vi "Flipping the Ramans for 3.0.vi"(0 "Folder Name":string, 1 "Name of File":string, 2 "Timepoints":dbl[](array[numeric]), 3 "Vx array":dbl, 4 "Vy array":dbl) -> ()   [LabVIEW 2015]
uses:
  <vilib>/Utility/file.llb/Read Delimited Spreadsheet (DBL).vi
  <vilib>/Utility/file.llb/Write Delimited Spreadsheet (DBL).vi
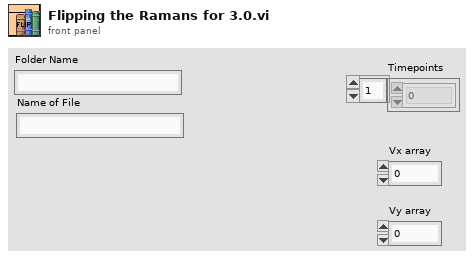
[diagram p1: front panel]
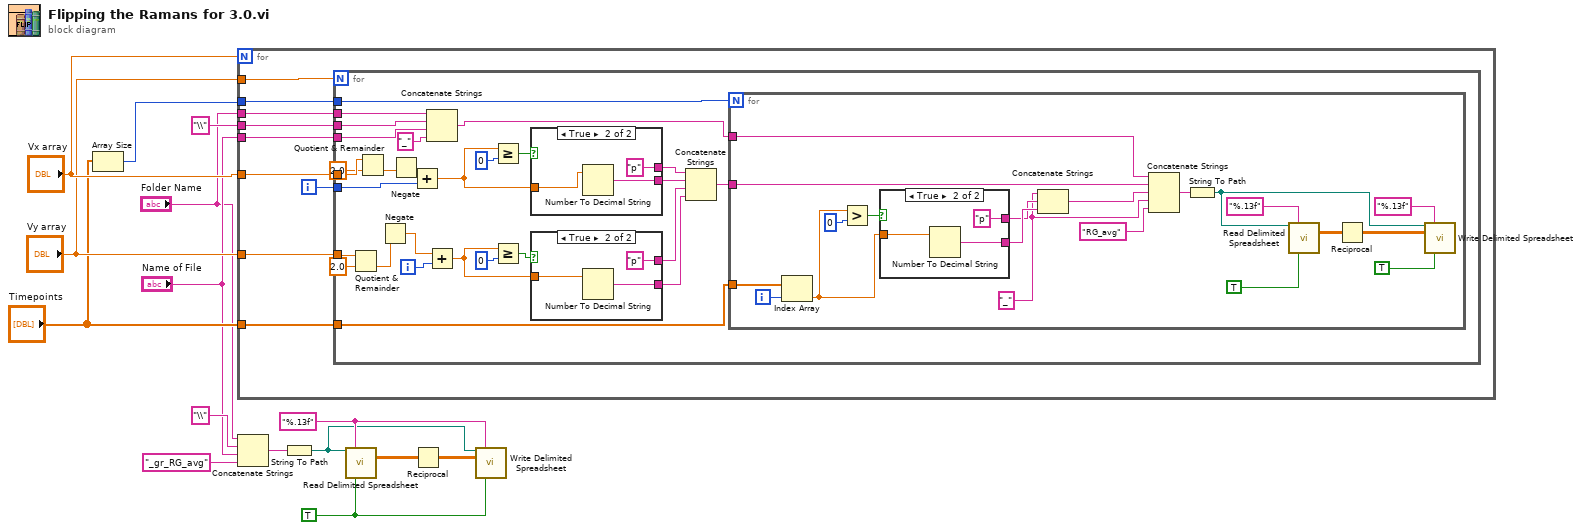
[diagram p0: block diagram]
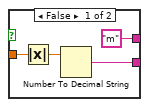
[diagram p2: hidden frame]
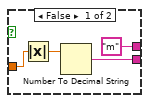
[diagram p3: hidden frame]
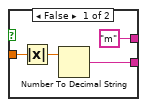
[diagram p4: hidden frame]
diagram:
  w3 = "%.13f" ("format (%.3f)")
  w2 = TRUE ("transpose? (F)")
  n1 = Array Size(array="Timepoints") -> (size(s)=w14:i32)
  n2 = for {
    N: "Vx array" -> [_]
    tunnel: "Name of File" -> [w24]
    tunnel: "\\" -> [w23]
    tunnel: "Folder Name" -> [w22]
    tunnel: "Vy array" -> [w21]
    tunnel: w14 -> [w20]
    tunnel: "Vx array" -> [w19]
    tunnel: "Vy array" -> [w17]
    tunnel: "Timepoints" -> [w16]
    i -> [w18]
    n3 = for {
      N: w21 -> [_]
      tunnel: w24 -> [w33]
      tunnel: w23 -> [w34]
      tunnel: w22 -> [w52]
      tunnel: w20 -> [w51]
      tunnel: w19 -> [w32]
      tunnel: w18 -> [w48]
      tunnel: w17 -> [w30]
      tunnel: w16 -> [w38]
      i -> [w43]
      n4 = Quotient & Remainder(x=w30, y=2.0) -> (floor(x/y)=w25:dbl)  [unwired: 1 out]
      n5 = Quotient & Remainder(x=w32, y=2.0) -> (floor(x/y)=w28:dbl)  [unwired: 1 out]
      n6 = Negate(x=w25) -> (-x=w26:dbl)
      n7 = Negate(x=w28) -> (-x=w27:dbl)
      n8 = Add(x=w27, y=w48) -> (x+y=w47:dbl)
      n9 = Concatenate Strings(w52, w34, w33, "_") -> (w36:string)
      n10 = Add(x=w26, y=w43) -> (x+y=w44:dbl)
      n11 = Greater Or Equal?(x=w47, y=0) -> (x >= y?=w49:bool)
      n12 = Greater Or Equal?(x=w44, y=0) -> (x >= y?=w46:bool)
      n13 = case shown="True" w49 {
        tunnel: ["m" "p"] -> w42
        tunnel: w47 -> [w62 w64]
        tunnel: [w60 w65] -> w41
        frame False {
          n14 = Absolute Value(x=w62) -> (abs(x)=w61:dbl)
          n15 = Number To Decimal String(number=w61) -> (decimal integer string=w60:string)  [unwired: 1 in]
        }
        frame True {
          n16 = Number To Decimal String(number=w64) -> (decimal integer string=w65:string)  [unwired: 1 in]
        }
      }
      n17 = case shown="True" w46 {
        tunnel: ["m" "p"] -> w40
        tunnel: w44 -> [w55 w57]
        tunnel: [w53 w58] -> w39
        frame False {
          n18 = Absolute Value(x=w55) -> (abs(x)=w54:dbl)
          n19 = Number To Decimal String(number=w54) -> (decimal integer string=w53:string)  [unwired: 1 in]
        }
        frame True {
          n20 = Number To Decimal String(number=w57) -> (decimal integer string=w58:string)  [unwired: 1 in]
        }
      }
      n21 = Concatenate Strings(w42, w41, w40, w39) -> (w35:string)
      n22 = for {
        N: w51 -> [_]
        tunnel: w38 -> [w83]
        tunnel: w36 -> [w74]
        tunnel: w35 -> [w73]
        i -> [w82]
        w72 = "_"
        n23 = Index Array(array=w83, index=w82) -> (element=w85:dbl)
        n24 = Greater?(x=w85, y=0) -> (0:w84:bool)
        n25 = case shown="True" w84 {
          tunnel: ["m" "p"] -> w80
          tunnel: w85 -> [w89 w91]
          tunnel: [w87 w92] -> w81
          frame False {
            n26 = Absolute Value(x=w89) -> (abs(x)=w88:dbl)
            n27 = Number To Decimal String(number=w88) -> (decimal integer string=w87:string)  [unwired: 1 in]
          }
          frame True {
            n28 = Number To Decimal String(number=w91) -> (decimal integer string=w92:string)  [unwired: 1 in]
          }
        }
        n29 = Concatenate Strings(w72, w80, w81) -> (w68:string)
        n30 = Concatenate Strings(w74, w73, w68, w72, "RG_avg") -> (w76:string)
        n31 = String To Path(string=w76) -> (path=w67:path)
        n32 = call-poly <vilib>:"Read Delimited Spreadsheet.vi"("file path (dialog if empty)"=w67, "format (%.3f)"="%.13f", "transpose? (F)"=TRUE) -> ("all rows"=w70:dbl[][])  [unwired: 7 in, 5 out]
        n33 = Reciprocal(x=w70) -> (1/x=w69:dbl[][])
        n34 = call-poly <vilib>:"Write Delimited Spreadsheet.vi"("file path (dialog if empty)"=w67, "format (%.3f)"="%.13f", "2D data"=w69, "transpose? (F)"=TRUE) -> ()  [unwired: 10 in, 2 out]
      }
    }
  }
  n35 = Concatenate Strings("Folder Name", "\\" ("string"), "Name of File", "_gr_RG_avg" ("string")) -> (w7:string)
  n36 = String To Path(string=w7) -> (path=w1:path)
  n37 = call-poly <vilib>:"Read Delimited Spreadsheet.vi"("file path (dialog if empty)"=w1, "format (%.3f)"=w3, "transpose? (F)"=w2) -> ("all rows"=w5:dbl[][])  [unwired: 7 in, 5 out]
  n38 = Reciprocal(x=w5) -> (1/x=w4:dbl[][])
  n39 = call-poly <vilib>:"Write Delimited Spreadsheet.vi"("file path (dialog if empty)"=w1, "format (%.3f)"=w3, "2D data"=w4, "transpose? (F)"=w2) -> ()  [unwired: 10 in, 2 out]
